vi "get_all_switches.vi"(8 "error in (no error)":errorcluster, 11 "Qtegra in":refnum<class "Qtegra.lvclass">) -> (0 "error out":errorcluster, 2 "actual switch states":bool[](array[boolean]), 3 "Qtegra out":refnum<class "Qtegra.lvclass">)   [LabVIEW 2017, in "Qtegra.lvclass"]
uses:
  Qtegra.lvclass
  \\Mac\Home/my data/University/Lamont/Software/LabView/MSControlSuite_Code/MSControl/Classes/Instrument/instrument.lvclass
  instrument.lvclass
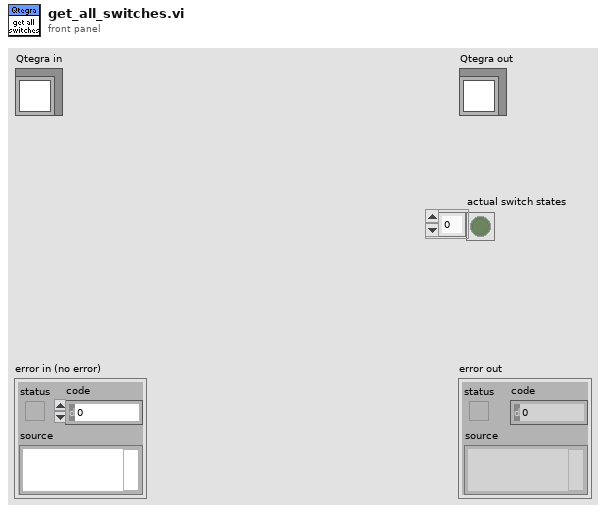
[diagram p1: front panel]
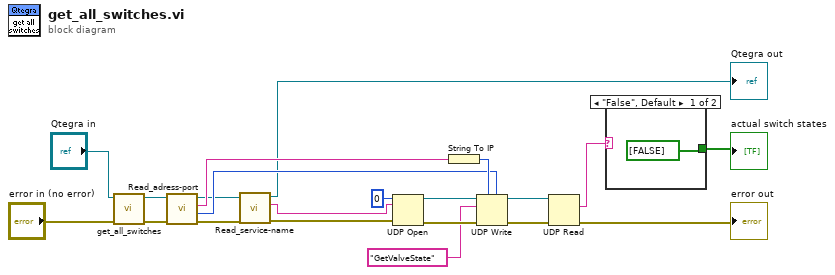
[diagram p0: block diagram]
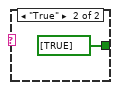
[diagram p2: hidden frame]
diagram:
  n1 = call-parent "get_all_switches.vi"("error in (no error)"="error in (no error)", "instrument in"="Qtegra in") -> ("error out"=w6:errorcluster, "instrument out"=w7:refnum<class "Qtegra.lvclass">)  [unwired: 7 in, 1 out]
  n2 = call "Read_adress-port.vi"("error in (no error)"=w6, "instrument in"=w7) -> ("error out"=w11:errorcluster, "port number"=w12:i32, "adress"=w19:string, "instrument out"=w10:refnum<class "Qtegra.lvclass">)  [unwired: 6 in]
  n3 = call-dynamic "Read_service-name.vi"("error in (no error)"=w11, "instrument in"=w10) -> ("error out"=w9:errorcluster, "service name"=w8:string, "instrument out"=→"Qtegra out":refnum<class "Qtegra.lvclass">)  [unwired: 7 in]
  n4 = UDP Open(8:w9, 10:w8, 11:u16 0 ("port")) -> (port=w15:refnum<k16>, 0:w16:errorcluster)  [unwired: 2 in, 1 out]
  n5 = String To IP(1:w19) -> (0:w18:u32)
  n6 = UDP Write(address=w18, port or service name=w12, connection ID=w15, data in="GetValveState", 8:w16) -> (error out=w13:errorcluster, 3:w14:refnum<k16>)  [unwired: 1 in]
  n7 = UDP Read(connection ID=w14, 8:w13) -> (data out=w2:string, error out=→"error out":errorcluster)  [unwired: 2 in, 3 out]
  n8 = case shown="\"False\", Default" w2 {
    tunnel: [bool[] [FALSE] bool[] [TRUE]] -> w1
    frame "False", Default {
    }
    frame "True" {
    }
  }
  "actual switch states" <- w1
